vi "Report Raw Data.vi"() -> (2 "Header Name":string[](array[string]))   [LabVIEW 2015]
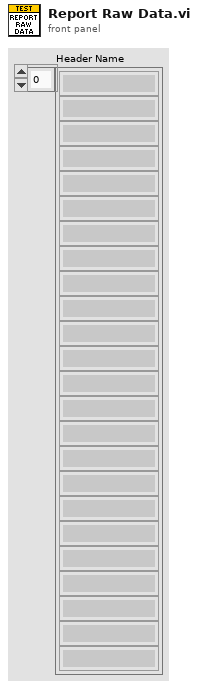
[diagram p1: front panel]
types:
  T1 = cluster{string, "element":string, "element 2":string, "element 3":string, "Load Min(N)":string, "Load Max(N)":string, "Dist Min(mm)":string, "Dist (mm)":string, "Dist Status":string, "Load Max(N) 2":string, "Dist Min(mm) 2":string, "Dist (mm) 2":string, "Dist Status 2":string, "Load Max(N) 3":string, "Dist Min(mm) 3":string, "Dist (mm) 3":string, "Dist Status 3":string}
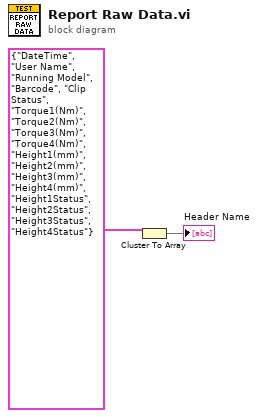
[diagram p0: block diagram]
diagram:
  n1 = Cluster To Array(cluster=T1 {"DateTime", "element"="User Name", "element 2"="Running Model", "element 3"="Barcode", "Load Min(N)"="Clip Status", "Load Max(N)"="Torque1(Nm)", "Dist Min(mm)"="Torque2(Nm)", "Dist (mm)"="Torque3(Nm)", "Dist Status"="Torque4(Nm)", "Load Max(N) 2"="Height1(mm)", "Dist Min(mm) 2"="Height2(mm)", "Dist (mm) 2"="Height3(mm)", "Dist Status 2"="Height4(mm)", "Load Max(N) 3"="Height1Status", "Dist Min(mm) 3"="Height2Status", "Dist (mm) 3"="Height3Status", "Dist Status 3"="Height4Status"} ("Sensor Data 2")) -> (array=→"Header Name":string[])
